vi "Creador de Fuente.vi"() -> ()   [LabVIEW 2010]
panel:
  in  "Abrir fuente":bool
  in  "Guardar":bool
  in  "stop":bool
  in  "Nueva fuente":bool
  out "ASCII (HEX)":u8 format="%x"
  out "ASCII (DEC)":u8
  in  "Letra":string="A"
  in  "Array booleano":bool[][](array[boolean])
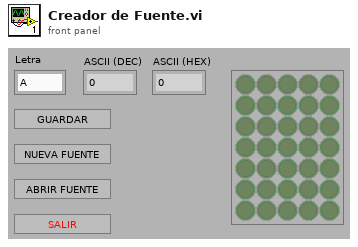
[diagram p1: front panel]
types:
  T1 = enum16{"open", "replace", "create", "open or create", "replace or create", "replace or create with confirmation"}
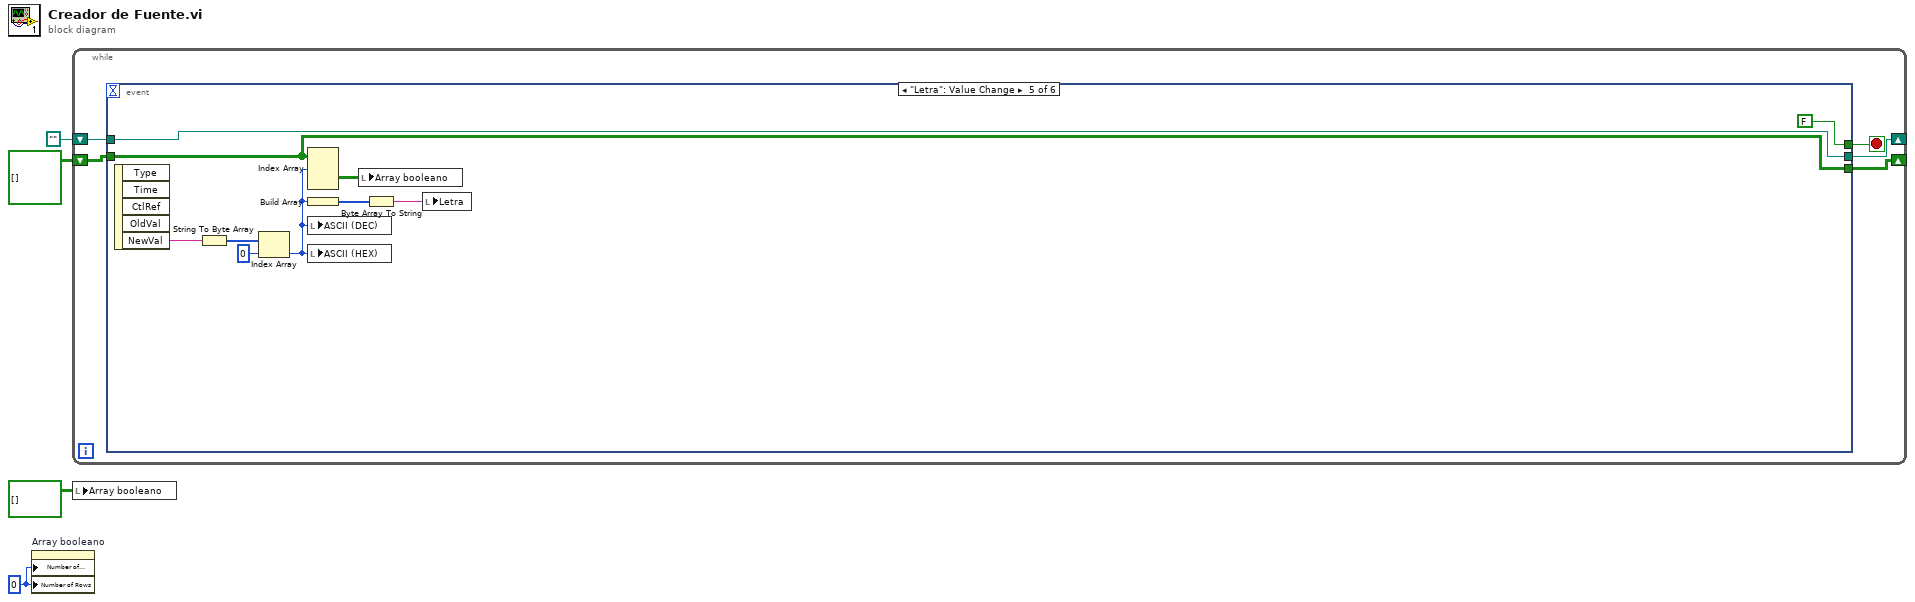
[diagram p0: block diagram]
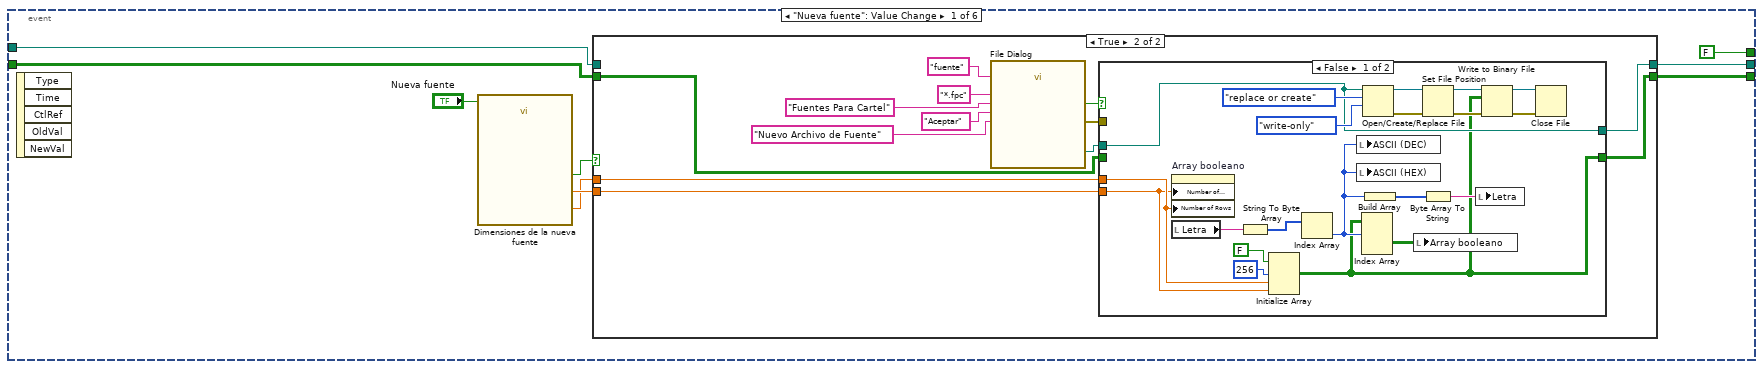
[diagram p2: hidden frame]
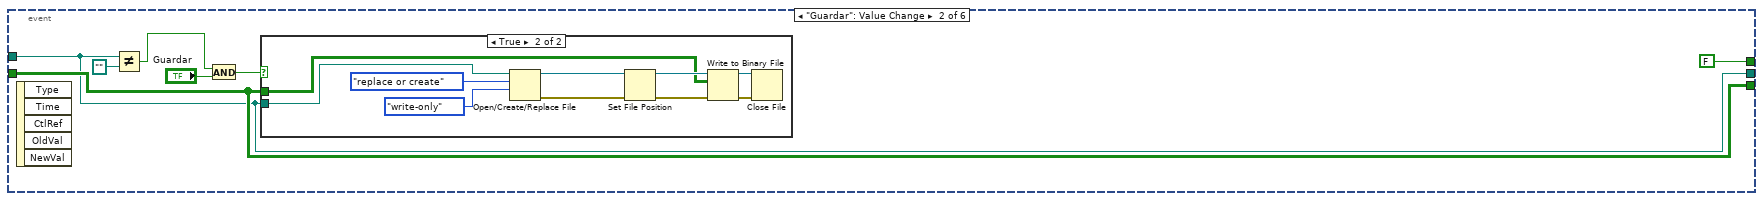
[diagram p5: hidden frame]
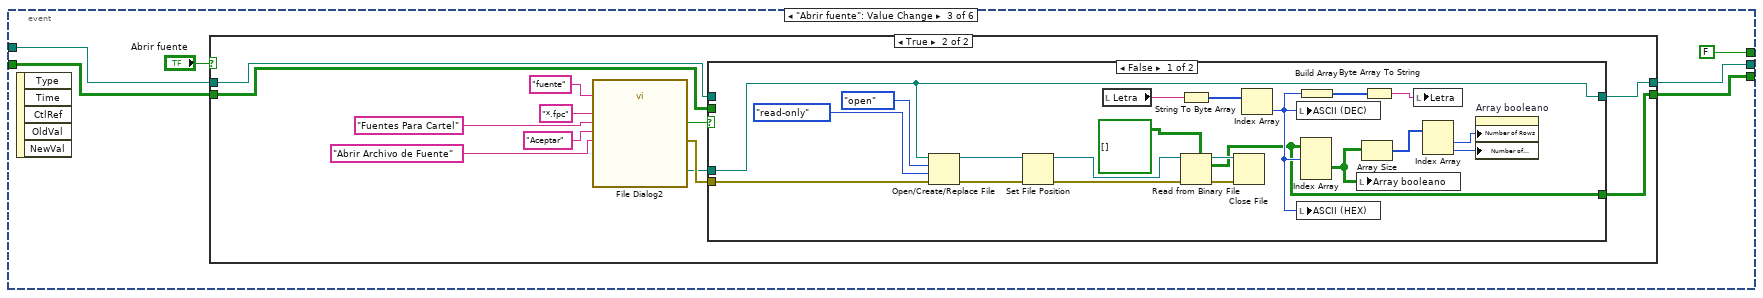
[diagram p7: hidden frame]
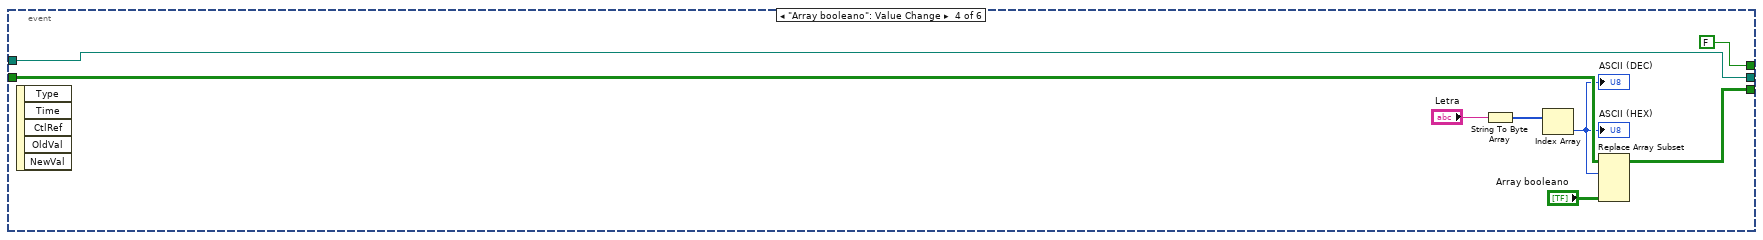
[diagram p10: hidden frame]
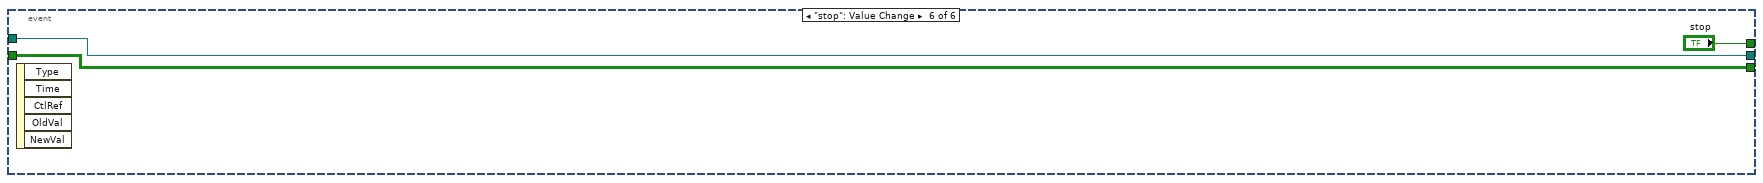
[diagram p11: hidden frame]
diagram:
  w1 = u32 0 ("Number of Columns")
  n1 = property on="Array booleano" class="Arr (strict)"("Number of Columns"=w1, "Number of Rows"=w1) -> ()  [unwired: 2 in, 2 out]
  n2 = while {
    shift-right: [w8] -> _
    shift-left: path "" -> [w7]
    shift-right: [w5] -> _
    shift-left: bool[][][] [] ("appended array") -> [w6]
    stop <- w9 stop-if-true
    n3 = event shown="[4] \"Letra\": Value Change" {
      selector: _ -> [_ _ _ _ _ _]
      dyn-events: _ -> [_ _ _ _ _ _]
      timeout: _ -> [_ _ _ _ _ _]
      tunnel: [FALSE ("stop") FALSE ("stop") FALSE ("stop") FALSE ("stop") FALSE ("stop") "stop"] -> w9
      tunnel: [w13 w59 w73 w120 w128 w135] -> w8
      tunnel: w7 -> [w12 w59 w74 w120 w128 w135]
      tunnel: w6 -> [w11 w62 w76 w119 w130 w134]
      tunnel: [w10 w62 w77 w118 w130 w134] -> w5
      event "Nueva fuente": Value Change {
        n4 = event-data() -> ()  [unwired: 1 in, 5 out]
        n5 = call "Dimensiones de la nueva fuente"("Enable"="Nueva fuente") -> ("Columnas"=w15:dbl, "Filas"=w14:dbl, "Crear"=w16:bool)  [unwired: 15 in, 1 out]
        n6 = case shown="True" w16 {
          tunnel: w15 -> [_ w27]
          tunnel: w14 -> [_ w26]
          tunnel: [w20 w21] -> w13
          tunnel: w12 -> [w20 _]
          tunnel: w11 -> [w19 w24]
          tunnel: [w19 w23] -> w10
          frame False {
          }
          frame True {
            n7 = call "File Dialog"("prompt"="Nuevo Archivo de Fuente", "button label"="Aceptar", "default name"="fuente", "pattern (all files)"="*.fpc", "pattern label"="Fuentes Para Cartel") -> ("selected path"=w22:path, "cancelled"=w28:bool, "error out"=w25:errorcluster)  [unwired: 7 in, 1 out]
            n8 = case shown="False" w28 {
              tunnel: w27 -> [w50 _]
              tunnel: w26 -> [w51 _]
              tunnel: w25 -> [_ _]
              tunnel: [w35 w55] -> w23
              tunnel: w24 -> [_ w55]
              tunnel: w22 -> [w41 w54]
              tunnel: [w41 w54] -> w21
              frame False {
                n9 = property on="Array booleano" class="Arr (strict)"("Number of Columns"=w50, "Number of Rows"=w51) -> ()  [unwired: 2 in, 2 out]
                n10 = local read "Letra"() -> (w34:string)
                n11 = String To Byte Array(string=w34) -> (unsigned byte array=w39:u8[])
                n12 = Initialize Array(FALSE, 256 ("dimension size"), w51, w50) -> (w35:bool[][][])
                n13 = Index Array(array=w39) -> (element=w36:u8)  [unwired: 1 in]
                n14 = local write "ASCII (DEC)"(w36) -> ()
                n15 = local write "ASCII (HEX)"(w36) -> ()
                n16 = Index Array(array=w35, index (dim 0)=w36) -> (element=w38:bool[][])  [unwired: 2 in]
                n17 = Open/Create/Replace File(file path (use dialog)=w41, operation (0:open)=T1."replace or create", access (0:read/write)=enum16{"read/write", "read-only", "write-only"}."write-only") -> (refnum out=w45:refnum<file>, error out=w46:errorcluster)  [unwired: 3 in, 1 out]
                n18 = Build Array(w36) -> (w40:u8[])
                n19 = local write "Array booleano"(w38) -> ()
                n20 = Set File Position(refnum=w45, error in=w46) -> (refnum out=w44:refnum<file>, error out=w47:errorcluster)  [unwired: 2 in]
                n21 = Byte Array To String(unsigned byte array=w40) -> (string=w37:string)
                n22 = local write "Letra"(w37) -> ()
                n23 = Write to Binary File(file (use dialog)=w44, data=w35, error in=w47) -> (refnum out=w42:refnum<file>, error out=w43:errorcluster)  [unwired: 3 in, 1 out]
                n24 = Close File(refnum=w42, error in=w43) -> ()  [unwired: 2 out]
              }
              frame True {
              }
            }
          }
        }
      }
      event "Guardar": Value Change {
        n25 = event-data() -> ()  [unwired: 1 in, 5 out]
        n26 = Not Equal?(x=w59, y=path "") -> (x != y?=w58:bool)
        n27 = And(x=w58, y="Guardar") -> (x .and. y?=w56:bool)
        n28 = case shown="True" w56 {
          tunnel: w59 -> [_ w72]
          tunnel: w62 -> [_ w65]
          frame False {
          }
          frame True {
            n29 = Open/Create/Replace File(file path (use dialog)=w72, operation (0:open)=T1."replace or create", access (0:read/write)=enum16{"read/write", "read-only", "write-only"}."write-only") -> (refnum out=w67:refnum<file>, error out=w68:errorcluster)  [unwired: 3 in, 1 out]
            n30 = Set File Position(refnum=w67, error in=w68) -> (refnum out=w66:refnum<file>, error out=w69:errorcluster)  [unwired: 2 in]
            n31 = Write to Binary File(file (use dialog)=w66, data=w65, error in=w69) -> (refnum out=w63:refnum<file>, error out=w64:errorcluster)  [unwired: 3 in, 1 out]
            n32 = Close File(refnum=w63, error in=w64) -> ()  [unwired: 2 out]
          }
        }
      }
      event "Abrir fuente": Value Change {
        n33 = event-data() -> ()  [unwired: 1 in, 5 out]
        n34 = case shown="True" "Abrir fuente" {
          tunnel: [w80 w84] -> w77
          tunnel: w76 -> [w80 w83]
          tunnel: w74 -> [w79 w81]
          tunnel: [w79 w82] -> w73
          frame False {
          }
          frame True {
            n35 = call "File Dialog2"("prompt"="Abrir Archivo de Fuente", "button label"="Aceptar", "default name"="fuente", "pattern (all files)"="*.fpc", "pattern label"="Fuentes Para Cartel") -> ("selected path"=w85:path, "cancelled"=w87:bool, "error out"=w86:errorcluster)  [unwired: 7 in, 1 out]
            n36 = case shown="False" w87 {
              tunnel: w86 -> [w113 _]
              tunnel: w85 -> [w103 _]
              tunnel: [w98 w115] -> w84
              tunnel: w83 -> [_ w115]
              tunnel: [w103 w114] -> w82
              tunnel: w81 -> [_ w114]
              frame False {
                n37 = Open/Create/Replace File(file path (use dialog)=w103, error in=w113, operation (0:open)=T1."open", access (0:read/write)=enum16{"read/write", "read-only", "write-only"}."read-only") -> (refnum out=w109:refnum<file>, error out=w110:errorcluster)  [unwired: 2 in, 1 out]
                n38 = Set File Position(refnum=w109, error in=w110) -> (refnum out=w107:refnum<file>, error out=w108:errorcluster)  [unwired: 2 in]
                n39 = local read "Letra"() -> (w97:string)
                n40 = String To Byte Array(string=w97) -> (unsigned byte array=w101:u8[])
                n41 = Read from Binary File(5:bool[][][] [] ("appended array"), 8:w108, 11:w107) -> (0:w105:errorcluster, 2:w98:bool[][][], 3:w106:refnum<file>)  [unwired: 3 in, 1 out]
                n42 = Close File(refnum=w106, error in=w105) -> ()  [unwired: 2 out]
                n43 = Index Array(array=w101) -> (element=w99:u8)  [unwired: 1 in]
                n44 = local write "ASCII (DEC)"(w99) -> ()
                n45 = local write "ASCII (HEX)"(w99) -> ()
                n46 = Index Array(array=w98, index (dim 0)=w99) -> (element=w96:bool[][])  [unwired: 2 in]
                n47 = Build Array(w99) -> (w102:u8[])
                n48 = local write "Array booleano"(w96) -> ()
                n49 = Array Size(array=w96) -> (size(s)=w95:i32[])
                n50 = Byte Array To String(unsigned byte array=w102) -> (string=w100:string)
                n51 = local write "Letra"(w100) -> ()
                n52 = Index Array(array=w95) -> (element #1=w94:i32, element #2=w93:i32)  [unwired: 2 in]
                n53 = property on="Array booleano" class="Arr (strict)"("Number of Rows"=w94, "Number of Columns"=w93) -> ()  [unwired: 2 in, 2 out]
              }
              frame True {
              }
            }
          }
        }
      }
      event "Array booleano": Value Change {
        n54 = event-data() -> ()  [unwired: 1 in, 5 out]
        n55 = String To Byte Array(string="Letra") -> (unsigned byte array=w123:u8[])
        n56 = Index Array(array=w123) -> (element=w116:u8)  [unwired: 1 in]
        "ASCII (DEC)" <- w116
        "ASCII (HEX)" <- w116
        n57 = Replace Array Subset(array=w119, new element="Array booleano", index (dim 0)=w116) -> (w118:bool[][][])  [unwired: 2 in]
      }
      event "Letra": Value Change {
        n58 = event-data() -> ("NewVal"=w127:string)  [unwired: 1 in, 4 out]
        n59 = String To Byte Array(string=w127) -> (unsigned byte array=w132:u8[])
        n60 = Index Array(array=w132, index=0) -> (element=w125:u8)
        n61 = Index Array(array=w130, index (dim 0)=w125) -> (element=w131:bool[][])  [unwired: 2 in]
        n62 = Build Array(w125) -> (w133:u8[])
        n63 = local write "ASCII (DEC)"(w125) -> ()
        n64 = local write "ASCII (HEX)"(w125) -> ()
        n65 = local write "Array booleano"(w131) -> ()
        n66 = Byte Array To String(unsigned byte array=w133) -> (string=w126:string)
        n67 = local write "Letra"(w126) -> ()
      }
      event "stop": Value Change {
        n68 = event-data() -> ()  [unwired: 1 in, 5 out]
      }
    }
  }
  n69 = local write "Array booleano"(bool[][] [] ("appended array")) -> ()
